vi "pulsed_counts.vi"(0 "commands":T1(array[cluster]) {"Time" format="%.3p"; "Op Code" items=["Continue", "Stop", "Loop", "End Loop", "JSR", "RTS", "Branch", "Long Delay", "Wait"]}) -> (4 "timetags":u32[](graph), 6 "triggers":u32[](array[numeric]), 15 "Error_out":errorcluster)   [LabVIEW 2018]
uses:
  <vilib>/DAQmx/read.llb/DAQmx Read (Counter 1D U32 1Chan NSamp).vi
  <vilib>/DAQmx/miscellaneous.llb/DAQmx Fill In Error Info.vi
panel:
  # "1"
  # "2"
  # "3"
  # "4"
  # "5"
  # "6"
  # "7"
  # "8"
  # "9"
  # "10"
  # "11"
  # "12"
  # "13"
  # "14"
  # "15"
  # "16"
  # "17"
  # "18"
  # "19"
  # "20"
  # "21"
  # "22"
  # "23"
  # "24"
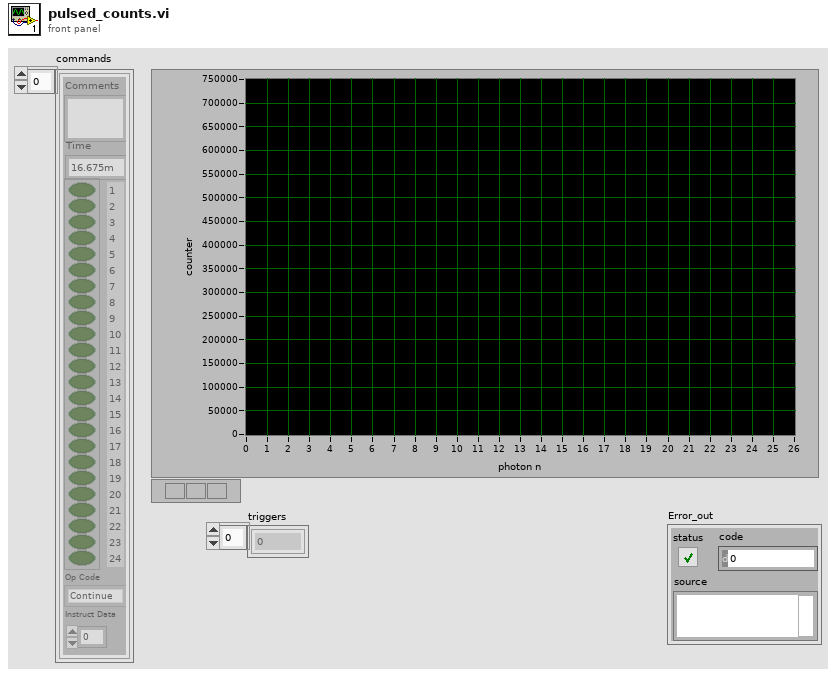
[diagram p1: front panel]
types:
  T1 = cluster{"Instruct Data":i32, "Op Code":i32, "Flags":bool[], "Comments":string, "Time":dbl}[]
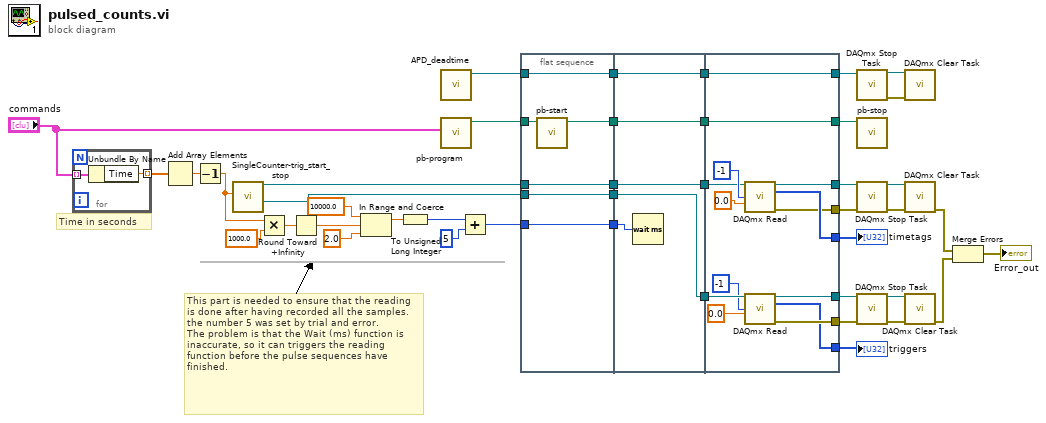
[diagram p0: block diagram]
diagram:
  # "Time in seconds"
  # "This part is needed to ensure that the reading is done after having recorded all the samples. the number 5 was set by trial and error. \nThe problem is that the Wait (ms) function is inaccurate, so it can triggers the reading\nfunction before the pulse sequences have\nfinished."
  n1 = for {
    tunnel: "commands" -> [w45] mode=indexing
    tunnel: [w44] -> w18 mode=indexing
    n2 = Unbundle By Name(w45) -> ("Time"=w44:dbl)
  }
  n3 = Add Array Elements(numeric array=w18) -> (sum=w17:dbl)
  n4 = Decrement(x=w17) -> (x-1=w14:dbl)
  n5 = call "SingleCounter-trig_start_stop.vi"("Duration_s"=w14) -> ("triggers_task"=w11:refnum<k21>, "APD_task"=w15:refnum<k21>)  [unwired: 7 in, 2 out]
  n6 = Multiply(x=w14, y=1000.0) -> (x*y=w21:dbl)
  n7 = Round Toward +Infinity(x=w21) -> (ceil(x): smallest int >= x=w20:dbl)
  n8 = In Range and Coerce(upper limit=10000.0, x=w20, lower limit=2.0) -> (coerced(x)=w38:dbl)  [unwired: 1 out]
  n9 = To Unsigned Long Integer(number=w38) -> (unsigned 32bit integer=w37:u32)
  n10 = call "APD_deadtime.vi"() -> ("filtered APD"=w32:refnum<k21>)  [unwired: 6 in, 1 out]
  n11 = call "pb-program.vi"("Commands"="commands") -> ("path out"=w27:path)  [unwired: 10 in]
  n12 = Add(x=w37, y=u32 5) -> (x+y=w2:u32)
  n13 = flat-sequence {
    tunnel: w32 -> [w49]
    tunnel: w2 -> [w50]
    tunnel: w15 -> [w51]
    tunnel: [w51] -> w30
    tunnel: [w50] -> w29
    tunnel: [w49] -> w28
    tunnel: w27 -> [w48]
    tunnel: [w47] -> w24
    tunnel: [w46] -> w12
    tunnel: w11 -> [w46]
    tunnel: [w56] -> w39
    tunnel: [w54] -> w33
    tunnel: w30 -> [w56]
    tunnel: w29 -> [w55]
    tunnel: w28 -> [w54]
    tunnel: [w53] -> w25
    tunnel: w24 -> [w53]
    tunnel: [w52] -> w13
    tunnel: w12 -> [w52]
    tunnel: [w69] -> w34
    tunnel: w39 -> [w68]
    tunnel: [w66] -> w31
    tunnel: w33 -> [w66]
    tunnel: [w65] -> w26
    tunnel: w25 -> [w65]
    tunnel: [w64] -> w23
    tunnel: [w63] -> w22
    tunnel: w13 -> [w62]
    tunnel: [w59] -> w8
    tunnel: [w58] -> w7
    tunnel: [w57] -> w3
    frame #0 {
      n14 = call "pb-start.vi"("path in"=w48) -> ("path out"=w47:path)  [unwired: 10 in]
    }
    frame #1 {
      n15 = Wait (ms)(milliseconds to wait=w55) -> ()  [unwired: 1 out]
    }
    frame #2 {
      n16 = call-poly <vilib>:"DAQmx Read.vi"("task/channels in"=w68, "number of samples per channel"=-1, "timeout"=0.0) -> ("task out"=w64:refnum<k21>, "data"=w69:u32[], "error out"=w63:errorcluster)  [unwired: 10 in]
      n17 = call-poly <vilib>:"DAQmx Read.vi"("task/channels in"=w62, "number of samples per channel"=-1, "timeout"=0.0) -> ("task out"=w59:refnum<k21>, "data"=w57:u32[], "error out"=w58:errorcluster)  [unwired: 10 in]
    }
  }
  n18 = call <vilib>:"DAQmx Stop Task.vi"("task/channels in"=w31) -> ("task out"=w41:refnum<k21>, "error out"=w40:errorcluster)  [unwired: 13 in]
  n19 = call "pb-stop.vi"("path in"=w26) -> ()  [unwired: 9 in, 2 out]
  n20 = call <vilib>:"DAQmx Stop Task.vi"("task/channels in"=w23, "error in"=w22) -> ("task out"=w43:refnum<k21>, "error out"=w42:errorcluster)  [unwired: 12 in]
  n21 = call <vilib>:"DAQmx Stop Task.vi"("task/channels in"=w8, "error in"=w7) -> ("task out"=w10:refnum<k21>, "error out"=w9:errorcluster)  [unwired: 12 in]
  n22 = call <vilib>:"DAQmx Clear Task.vi"("task in"=w41, "error in"=w40) -> ()  [unwired: 13 in, 1 out]
  n23 = call <vilib>:"DAQmx Clear Task.vi"("task in"=w43, "error in"=w42) -> ("error out"=w5:errorcluster)  [unwired: 13 in]
  n24 = call <vilib>:"DAQmx Clear Task.vi"("task in"=w10, "error in"=w9) -> ("error out"=w6:errorcluster)  [unwired: 13 in]
  n25 = Merge Errors(w5, w6) -> (→"Error_out":errorcluster)
  "timetags" <- w34
  "triggers" <- w3
